vi "Get Components.vi"(8 "error in":errorcluster, 11 "GPIB in":refnum<class "GPIB Board Design.lvclass">) -> (0 "error out":errorcluster, 2 "components":refnum<class "Component.lvclass">[](array[class]), 3 "GPIB out":refnum<class "GPIB Board Design.lvclass">)   [LabVIEW 2023, in "GPIB Board Design.lvclass"]
doc: "Get an array of components for the board."
uses:
  GPIB Board Design.lvclass
  Component/Component.lvclass
  ADConverter/AD Converter.lvclass
  c:/dev/_r/4/eng/lv-core/lvpostprocessingd/lv_mc_x86_64/dist_i386/examples/Object-Oriented Programming/Board Testing/Object Design/Component/Component.lvclass
  DAConverter/DA Converter.lvclass
  FPGAChip/FPGA Chip.lvclass
  Board/Component Orientation and Position.ctl
  Resistor/Resistor.lvclass
  Board/Board Design.lvclass
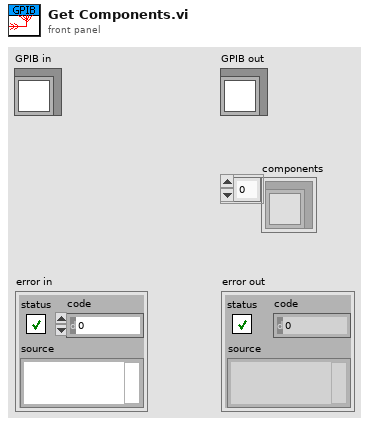
[diagram p1: front panel]
types:
  T1 = typedef "Board Design.lvclass/Component Orientation and Position.ctl" = cluster{"row":i16, "column":i16, "landscape?":bool}
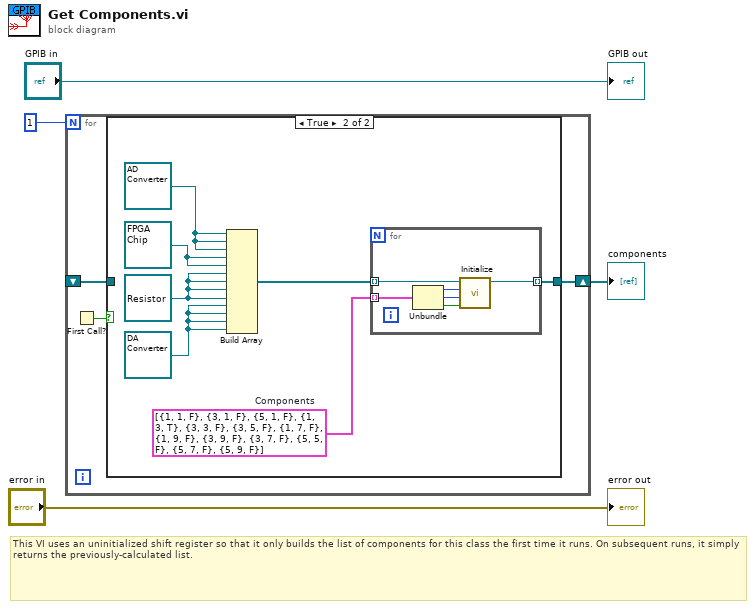
[diagram p0: block diagram]
diagram:
  # "This VI uses an uninitialized shift register so that it only builds the list of components for this class the first time it runs. On subsequent runs, it simply returns the previously-calculated list."
  n1 = for {
    N: 1 -> [_]
    shift-right: [w7] -> w2
    shift-left: _ -> [w5]
    n2 = First Call?() -> (First Call?: T/F=w6:bool)
    n3 = case shown="True" w6 {
      tunnel: [w8 w15] -> w7
      tunnel: w5 -> [w8 _]
      frame False {
      }
      frame True {
        w11 = refnum<class "Resistor.lvclass"> refnum ("Resistor.lvclass")
        w9 = T1[] [{"row"=1, "column"=1, "landscape?"=FALSE}, {"row"=3, "column"=1, "landscape?"=FALSE}, {"row"=5, "column"=1, "landscape?"=FALSE}, {"row"=1, "column"=3, "landscape?"=TRUE}, {"row"=3, "column"=3, "landscape?"=FALSE}, {"row"=3, "column"=5, "landscape?"=FALSE}, {"row"=1, "column"=7, "landscape?"=FALSE}, {"row"=1, "column"=9, "landscape?"=FALSE}, {"row"=3, "column"=9, "landscape?"=FALSE}, {"row"=3, "column"=7, "landscape?"=FALSE}, {"row"=5, "column"=5, "landscape?"=FALSE}, {"row"=5, "column"=7, "landscape?"=FALSE}, {"row"=5, "column"=9, "landscape?"=FALSE}]  # Components
        w14 = refnum<class "FPGA Chip.lvclass"> refnum ("FPGA Chip.lvclass")
        w10 = refnum<class "DA Converter.lvclass"> refnum ("DA Converter.lvclass")
        w12 = refnum<class "AD Converter.lvclass"> refnum ("AD Converter.lvclass")
        n4 = Build Array(w12, w12, w12, w14, w14, w11, w11, w11, w11, w10, w10, w10, w10) -> (w13:refnum<class "Component.lvclass">[])
        n5 = for {
          tunnel: w13 -> [w20] mode=indexing
          tunnel: [w21] -> w15 mode=indexing
          tunnel: w9 -> [w19] mode=indexing
          n6 = Unbundle(w19) -> ("row"=w18:i16, "column"=w17:i16, "landscape?"=w16:bool)
          n7 = call "Initialize.vi"("landscape?"=w16, "column"=w17, "row"=w18, "Component.lvclass in"=w20) -> ("Component.lvclass out"=w21:refnum<class "Component.lvclass">)  [unwired: 7 in]
        }
      }
    }
  }
  "components" <- w2
  "error out" <- "error in"
  "GPIB out" <- "GPIB in"
